vi "Read Action.vi"(8 "error in (no error)":errorcluster, 11 "Dot Settings in":refnum<class "Dot Settings.lvclass">) -> (0 "error out":errorcluster, 2 "Action":T1, 3 "Dot Settings out":refnum<class "Dot Settings.lvclass">)   [LabVIEW 2019, in "Dot Settings.lvclass"]
uses:
  Dot Settings.lvclass
  TypeDefs/Action.ctl
  Dot Settings.lvclass/Dot Settings.ctl
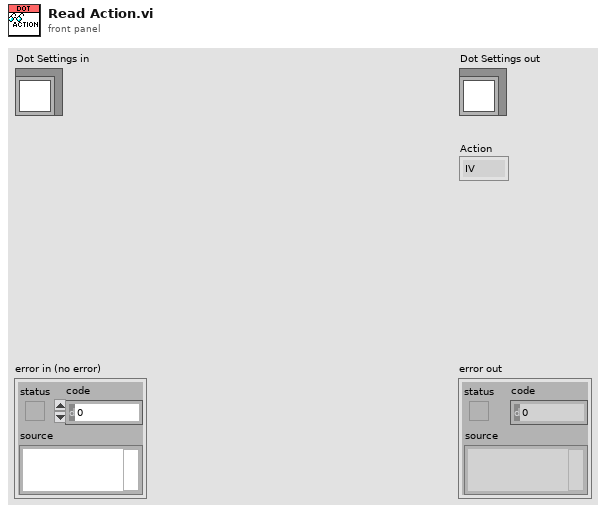
[diagram p1: front panel]
types:
  T1 = typedef "Dot Settings.lvclass/Action.ctl" = enum16{"IV", "QD"}
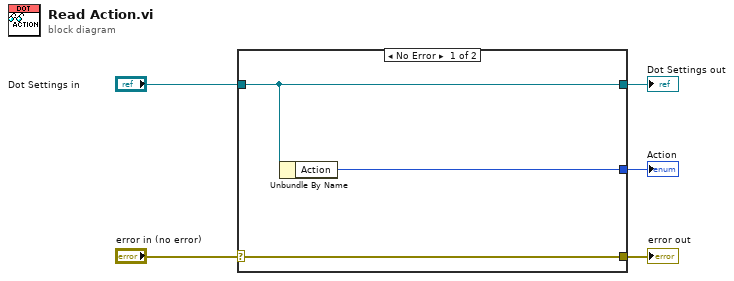
[diagram p0: block diagram]
diagram:
  n1 = case shown="No Error" "error in (no error)" {
    selector: "error in (no error)" -> [w8 w9]
    tunnel: [w8 w9] -> w4
    tunnel: [w7 w10] -> w2
    tunnel: "Dot Settings in" -> [w7 w10]
    tunnel: [w6 _] -> w1
    frame No Error {
      n2 = Unbundle By Name(w7) -> ("Action"=w6:T1)
    }
    frame Error {
    }
  }
  "error out" <- w4
  "Dot Settings out" <- w2
  "Action" <- w1
